vi "read responses.vi"(8 "error in":errorcluster, 11 "profibus reference":T3) -> (0 "error out":errorcluster, 2 "responses":T1[](array[typedef]), 3 "profibus reference out":T3)   [LabVIEW 2013, in "dynamic profibus.lvlib"]
uses:
  dynamic profibus.lvlib
  fpga reference.ctl
  full response.ctl
  profibus master transmit header.ctl
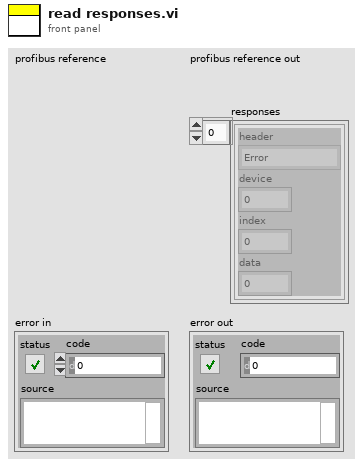
[diagram p1: front panel]
types:
  T1 = typedef "dynamic profibus.lvlib/full response.ctl" = cluster{"header":T2, "device":u8, "index":u8, "data":u8}
  T2 = typedef "dynamic profibus.lvlib/profibus master transmit header.ctl" = enum8{"Error", "Input", "Diagnostic", "input size", "output size"}
  T3 = typedef "dynamic profibus.lvlib/fpga reference.ctl" = refnum<k20>
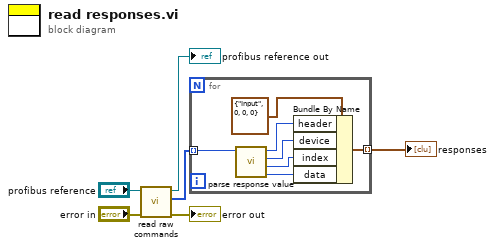
[diagram p0: block diagram]
diagram:
  n1 = call "read raw commands.vi"("error in"="error in", "profibus reference"="profibus reference") -> ("error out"=→"error out":errorcluster, "Data"=w2:u32[], "profibus reference out"=→"profibus reference out":T3)  [unwired: 7 in]
  n2 = for {
    tunnel: w2 -> [w13] mode=indexing
    tunnel: [w7] -> w1 mode=indexing
    n3 = call "parse response value.vi"("Element"=w13) -> ("data"=w8:u8, "index"=w11:u8, "device"=w10:u8, "header"=w9:T2)  [unwired: 7 in]
    n4 = Bundle By Name(cluster=T1 {"header"=enum."Input", "device"=0, "index"=0, "data"=0} ("command"), "header"=w9, "device"=w10, "index"=w11, "data"=w8) -> (w7:T1)
  }
  "responses" <- w1
